vi "Channel Overlap.vi"(7 "error source vi name":string, 8 "error in (no error)":errorcluster, 10 "channel block 2":T1 {"string descriptor"."buffer offset" format="%d bytes"; "engine descriptor"."buffer offset" format="%d bytes"}, 11 "channel block 1":T1 {"string descriptor"."buffer offset" format="%d bytes"; "engine descriptor"."buffer offset" format="%d bytes"}) -> (0 "error out":errorcluster)   [LabVIEW 2017, in "DSF Core.lvlib" / "Configuration Session.lvclass"]
uses:
  Configuration Session.lvclass
  Controls/DSF Engine Channel Configuration.ctl
  Controls/DSF Channel Buffer Descriptor.ctl
  Controls/DSF Data Type.ctl
  <vilib>/NI/Memory Manager/VIs/Source.Write.Scalar.Base10 (U64).vi
  Shared/VIs/Sizeof.vi
  Shared/Constants/Constants.vi
  Shared/Constants/Engine Library Name.vi
  <vilib>/NI/Memory Manager/VIs/Error Cluster.Set VI Source.vi
  <vilib>/NI/Memory Manager/VIs/Error Cluster.Set Code.vi
  <vilib>/NI/Memory Manager/VIs/Error Cluster.Set Status.vi
  <vilib>/NI/Memory Manager/VIs/New Error Cluster Constant.vi
  <vilib>/NI/Memory Manager/VIs/New Error Cluster Constant (512B).vi
  Configuration Error Info.vi
  Shared/Constants/Base Error Code.vi
  Shared/Constants/Error Offset (Configuration).vi
  <vilib>/NI/Memory Manager/Static Error Handling.lvlib
  DSF Core.lvlib
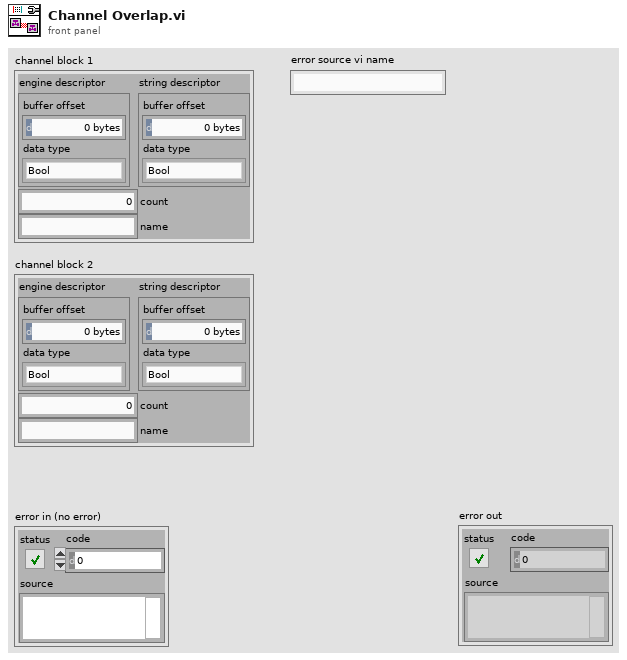
[diagram p1: front panel]
types:
  T1 = typedef "DSF Core.lvlib/DSF Engine Channel Configuration.ctl" = cluster{"engine descriptor":T2, "string descriptor":T2, "count":u64, "name":string}
  T2 = typedef "DSF Core.lvlib/DSF Channel Buffer Descriptor.ctl" = cluster{"buffer offset":u64, "data type":T3}
  T3 = typedef "DSF Core.lvlib/DSF Data Type.ctl" = enum8{"Bool", "SGL", "DBL", "I8", "I16", "I32", "I64", "U8", "U16", "U32", "U64"}
  T4 = enum16{"Channel Overlap", "Invalid Engine Offset"}
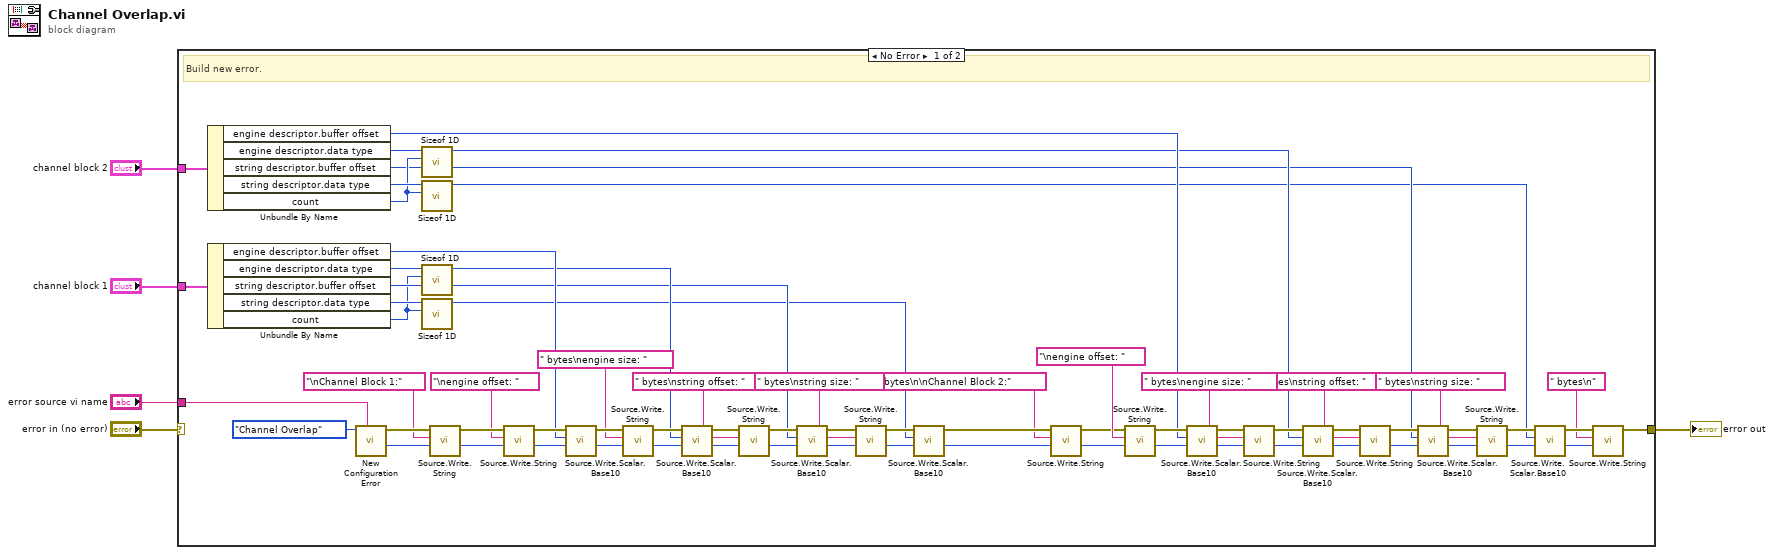
[diagram p0: block diagram]
diagram:
  n1 = case shown="No Error" "error in (no error)" {
    selector: "error in (no error)" -> [_ w74]
    tunnel: [w7 w74] -> w4
    tunnel: "error source vi name" -> [w72 _]
    tunnel: "channel block 1" -> [w69 _]
    tunnel: "channel block 2" -> [w62 _]
    frame No Error {
      # "Build new error."
      n2 = Unbundle By Name(w62) -> ("engine descriptor.buffer offset"=w14:u64, "engine descriptor.data type"=w39:T3, "string descriptor.buffer offset"=w12:u64, "string descriptor.data type"=w38:T3, "count"=w37:u64)
      n3 = Unbundle By Name(w69) -> ("engine descriptor.buffer offset"=w61:u64, "engine descriptor.data type"=w58:T3, "string descriptor.buffer offset"=w48:u64, "string descriptor.data type"=w47:T3, "count"=w46:u64)
      n4 = call "New Configuration Error.vi"("error source vi name"=w72, "configuration error"=T4."Channel Overlap") -> ("new offset"=w70:i32, "error out"=w71:errorcluster)  [unwired: 8 in]
      n5 = call "Sizeof 1D.vi"("count"=w37, "data type"=w39) -> ("size in bytes"=w13:u64)  [unwired: 9 in]
      n6 = call "Sizeof 1D.vi"("count"=w37, "data type"=w38) -> ("size in bytes"=w11:u64)  [unwired: 9 in]
      n7 = call "Sizeof 1D.vi"("count"=w46, "data type"=w58) -> ("size in bytes"=w54:u64)  [unwired: 9 in]
      n8 = call "Sizeof 1D.vi"("count"=w46, "data type"=w47) -> ("size in bytes"=w40:u64)  [unwired: 9 in]
      n9 = call <vilib>:"Source.Write.String.vi"("offset"=w70, "string"="\nChannel Block 1:", "error in"=w71) -> ("new offset"=w65:i32, "error out"=w67:errorcluster)  [unwired: 7 in]
      n10 = call <vilib>:"Source.Write.String.vi"("offset"=w65, "string"="\nengine offset: ", "error in"=w67) -> ("new offset"=w63:i32, "error out"=w64:errorcluster)  [unwired: 7 in]
      n11 = call-poly <vilib>:"Source.Write.Scalar.Base10.vi"("offset"=w63, "value"=w61, "error in"=w64) -> ("new offset"=w59:i32, "error out"=w60:errorcluster)  [unwired: 7 in]
      n12 = call <vilib>:"Source.Write.String.vi"("offset"=w59, "string"=" bytes\nengine size: ", "error in"=w60) -> ("new offset"=w55:i32, "error out"=w56:errorcluster)  [unwired: 7 in]
      n13 = call-poly <vilib>:"Source.Write.Scalar.Base10.vi"("offset"=w55, "value"=w54, "error in"=w56) -> ("new offset"=w52:i32, "error out"=w53:errorcluster)  [unwired: 7 in]
      n14 = call <vilib>:"Source.Write.String.vi"("offset"=w52, "string"=" bytes\nstring offset: ", "error in"=w53) -> ("new offset"=w49:i32, "error out"=w50:errorcluster)  [unwired: 7 in]
      n15 = call-poly <vilib>:"Source.Write.Scalar.Base10.vi"("offset"=w49, "value"=w48, "error in"=w50) -> ("new offset"=w42:i32, "error out"=w43:errorcluster)  [unwired: 7 in]
      n16 = call <vilib>:"Source.Write.String.vi"("offset"=w42, "string"=" bytes\nstring size: ", "error in"=w43) -> ("new offset"=w45:i32, "error out"=w44:errorcluster)  [unwired: 7 in]
      n17 = call-poly <vilib>:"Source.Write.Scalar.Base10.vi"("offset"=w45, "value"=w40, "error in"=w44) -> ("new offset"=w15:i32, "error out"=w16:errorcluster)  [unwired: 7 in]
      n18 = call <vilib>:"Source.Write.String.vi"("offset"=w15, "string"=" bytes\n\nChannel Block 2:", "error in"=w16) -> ("new offset"=w19:i32, "error out"=w17:errorcluster)  [unwired: 7 in]
      n19 = call <vilib>:"Source.Write.String.vi"("offset"=w19, "string"="\nengine offset: ", "error in"=w17) -> ("new offset"=w21:i32, "error out"=w20:errorcluster)  [unwired: 7 in]
      n20 = call-poly <vilib>:"Source.Write.Scalar.Base10.vi"("offset"=w21, "value"=w14, "error in"=w20) -> ("new offset"=w23:i32, "error out"=w22:errorcluster)  [unwired: 7 in]
      n21 = call <vilib>:"Source.Write.String.vi"("offset"=w23, "string"=" bytes\nengine size: ", "error in"=w22) -> ("new offset"=w26:i32, "error out"=w25:errorcluster)  [unwired: 7 in]
      n22 = call-poly <vilib>:"Source.Write.Scalar.Base10.vi"("offset"=w26, "value"=w13, "error in"=w25) -> ("new offset"=w28:i32, "error out"=w27:errorcluster)  [unwired: 7 in]
      n23 = call <vilib>:"Source.Write.String.vi"("offset"=w28, "string"=" bytes\nstring offset: ", "error in"=w27) -> ("new offset"=w31:i32, "error out"=w30:errorcluster)  [unwired: 7 in]
      n24 = call-poly <vilib>:"Source.Write.Scalar.Base10.vi"("offset"=w31, "value"=w12, "error in"=w30) -> ("new offset"=w35:i32, "error out"=w34:errorcluster)  [unwired: 7 in]
      n25 = call <vilib>:"Source.Write.String.vi"("offset"=w35, "string"=" bytes\nstring size: ", "error in"=w34) -> ("new offset"=w32:i32, "error out"=w33:errorcluster)  [unwired: 7 in]
      n26 = call-poly <vilib>:"Source.Write.Scalar.Base10.vi"("offset"=w32, "value"=w11, "error in"=w33) -> ("new offset"=w9:i32, "error out"=w8:errorcluster)  [unwired: 7 in]
      n27 = call <vilib>:"Source.Write.String.vi"("offset"=w9, "string"=" bytes\n", "error in"=w8) -> ("error out"=w7:errorcluster)  [unwired: 7 in, 1 out]
    }
    frame Error {
      # "Incoming error. Pass through."
    }
  }
  "error out" <- w4
